vi "Write Data File.vi"(8 "error in (no error)":errorcluster, 10 "Write Data File Arguments":T1, 11 "Test Log in":refnum<class "Test Log.lvclass">) -> (0 "error out":errorcluster, 2 "Relative Path":string, 3 "Test Log out":refnum<class "Test Log.lvclass">)   [LabVIEW 2015, in "Test Log.lvclass"]
uses:
  Test Log.lvclass
  Typedefs/Write Data File Arguments.ctl
  Typedefs/FAMT Typedefs.lvlib
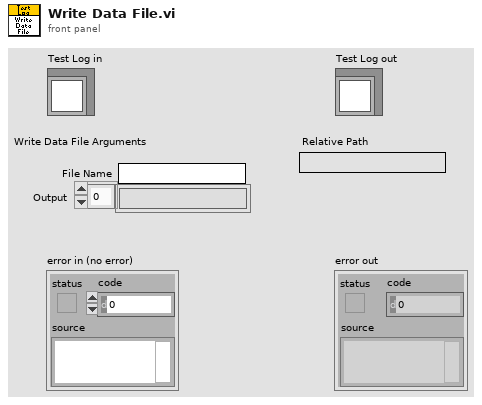
[diagram p1: front panel]
types:
  T1 = typedef "FAMT Typedefs.lvlib/Write Data File Arguments.ctl" = cluster{"File Name":string, "Output":string[]}
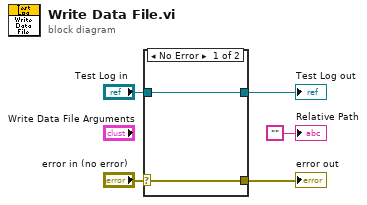
[diagram p0: block diagram]
diagram:
  n1 = case shown="No Error" "error in (no error)" {
    selector: "error in (no error)" -> [w6 w9]
    tunnel: [w6 w9] -> w5
    tunnel: [w7 w8] -> w3
    tunnel: "Test Log in" -> [w7 w8]
    frame No Error {
    }
    frame Error {
    }
  }
  "error out" <- w5
  "Test Log out" <- w3
  "Relative Path" <- ""
